vi "EXCOM_25_no_count.vi"(0 "VISA resource name":refnum<visa-resource-name>, 4 "error in":errorcluster) -> (5 "OK Done":bool, 6 "HA":dbl format="%<%H:%M:%S%0u>t", 7 "Q String":string, 8 "RA":dbl format="%<%H:%M:%S%0u>t", 9 "Rotateur":dbl format="%.2f", 10 "DEC":dbl format="%<%H:%M:%S%0u>t", 11 "Dome":dbl format="%.2f", 12 "Epoque":dbl format="%.2f", 13 "Focus":dbl format="%.2f", 14 "VISA resource name dup":refnum<visa-resource-name>, 15 "Masse d'air":dbl format="%.2f", 16 "Temps Sidéral":dbl format="%<%H:%M:%S%0u>t", 17 "Temps Universel":dbl format="%<%H:%M:%S%0u>t", 18 "Année":dbl format="%.2f", 19 "error out":errorcluster)   [LabVIEW 2011]
panel:
  # "3 = COM4"
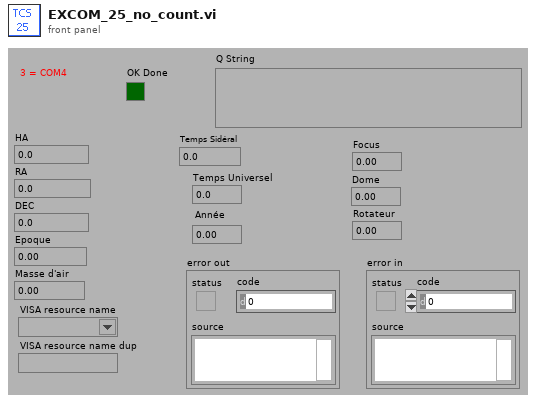
[diagram p1: front panel]
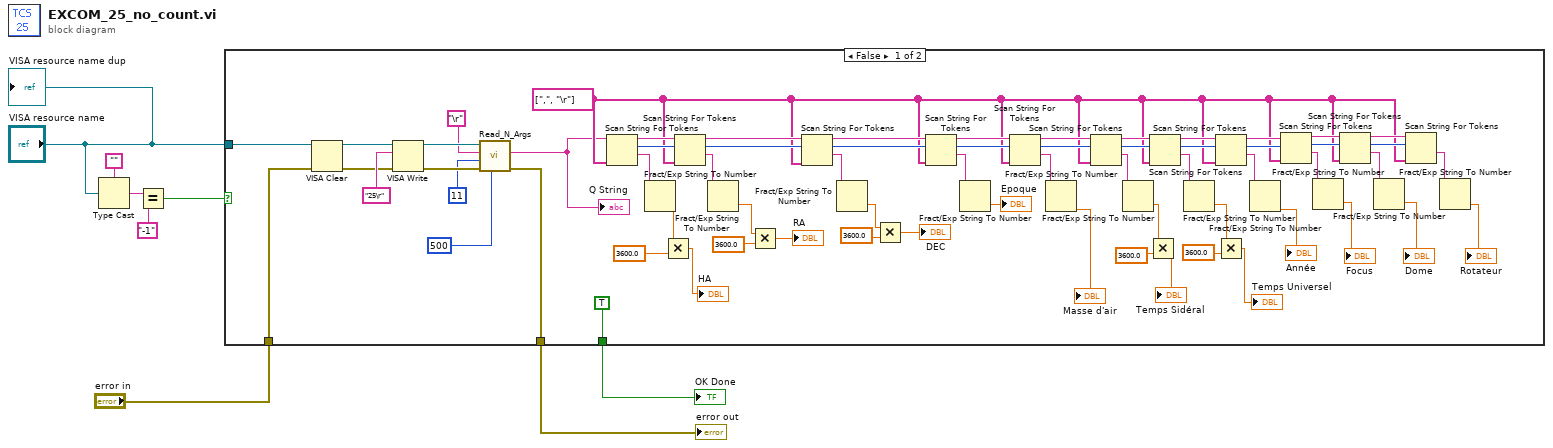
[diagram p0: block diagram]
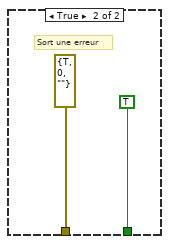
[diagram p2: hidden frame]
diagram:
  n1 = Type Cast(type="", x="VISA resource name") -> (*(type *) &x=w7:string)
  n2 = Equal?(x=w7, y="-1") -> (x = y?=w5:bool)
  n3 = case shown="False" w5 {
    tunnel: "VISA resource name" -> [w12 _]
    tunnel: [TRUE ("OK Done") TRUE ("OK Done")] -> w3
    tunnel: [w19 errorcluster {"status"=TRUE, "code"=0, "source"=""} ("error out")] -> w2
    tunnel: "error in" -> [w10 _]
    frame False {
      w23 = string[] [",", "\r"] ("delimiters (\\s,\\t,\\r,\\n)")
      n4 = VISA Clear(VISA resource name=w12, error in (no error)=w10) -> (VISA resource name out=w11:refnum<visa-resource-name>, error out=w9:errorcluster)
      n5 = VISA Write(VISA resource name=w11, write buffer="25\r" ("String to Send"), error in (no error)=w9) -> (VISA resource name out=w17:refnum<visa-resource-name>, error out=w18:errorcluster)  [unwired: 1 out]
      n6 = call "Read_N_Args.vi"("Delay (ms)"=u32 500, "Error IN"=w18, "Nb_Args"=11, "Arg_Char"="\r", "VRN IN"=w17) -> ("Error OUT"=w19:errorcluster, "Answer"=w20:string)  [unwired: 3 in, 2 out]
      "Q String" <- w20
      n7 = Scan String For Tokens(6:w23, 9:w20) -> (1:w66:string, 2:w67:i32, 3:w68:string)  [unwired: 4 in, 1 out]
      n8 = Fract/Exp String To Number(string=w66) -> (number=w65:dbl)  [unwired: 3 in, 1 out]
      n9 = Multiply(x=w65, y=3600.0) -> (x*y=→"HA":dbl)
      n10 = Scan String For Tokens(6:w23, 8:w67, 9:w68) -> (1:w24:string, 2:w70:i32, 3:w69:string)  [unwired: 3 in, 1 out]
      n11 = Fract/Exp String To Number(string=w24) -> (number=w57:dbl)  [unwired: 3 in, 1 out]
      n12 = Multiply(x=w57, y=3600.0) -> (x*y=→"RA":dbl)
      n13 = Scan String For Tokens(6:w23, 8:w70, 9:w69) -> (1:w60:string, 2:w72:i32, 3:w71:string)  [unwired: 3 in, 1 out]
      n14 = Fract/Exp String To Number(string=w60) -> (number=w55:dbl)  [unwired: 3 in, 1 out]
      n15 = Multiply(x=w55, y=3600.0) -> (x*y=→"DEC":dbl)
      n16 = Scan String For Tokens(6:w23, 8:w72, 9:w71) -> (1:w59:string, 2:w74:i32, 3:w73:string)  [unwired: 3 in, 1 out]
      n17 = Fract/Exp String To Number(string=w59) -> (number=→"Epoque":dbl)  [unwired: 3 in, 1 out]
      n18 = Scan String For Tokens(6:w23, 8:w74, 9:w73) -> (1:w58:string, 2:w26:i32, 3:w45:string)  [unwired: 3 in, 1 out]
      n19 = Fract/Exp String To Number(string=w58) -> (number=→"Masse d'air":dbl)  [unwired: 3 in, 1 out]
      n20 = Scan String For Tokens(6:w23, 8:w26, 9:w45) -> (1:w50:string, 2:w48:i32, 3:w49:string)  [unwired: 3 in, 1 out]
      n21 = Fract/Exp String To Number(string=w50) -> (number=w53:dbl)  [unwired: 3 in, 1 out]
      n22 = Multiply(x=w53, y=3600.0) -> (x*y=→"Temps Sidéral":dbl)
      n23 = Scan String For Tokens(6:w23, 8:w48, 9:w49) -> (1:w51:string, 2:w46:i32, 3:w47:string)  [unwired: 3 in, 1 out]
      n24 = Fract/Exp String To Number(string=w51) -> (number=w54:dbl)  [unwired: 3 in, 1 out]
      n25 = Scan String For Tokens(6:w23, 8:w46, 9:w47) -> (1:w52:string, 2:w25:i32, 3:w35:string)  [unwired: 3 in, 1 out]
      n26 = Multiply(x=w54, y=3600.0) -> (x*y=→"Temps Universel":dbl)
      n27 = Fract/Exp String To Number(string=w52) -> (number=→"Année":dbl)  [unwired: 3 in, 1 out]
      n28 = Scan String For Tokens(6:w23, 8:w25, 9:w35) -> (1:w38:string, 2:w40:i32, 3:w39:string)  [unwired: 3 in, 1 out]
      n29 = Fract/Exp String To Number(string=w38) -> (number=→"Focus":dbl)  [unwired: 3 in, 1 out]
      n30 = Scan String For Tokens(6:w23, 8:w40, 9:w39) -> (1:w37:string, 2:w42:i32, 3:w41:string)  [unwired: 3 in, 1 out]
      n31 = Fract/Exp String To Number(string=w37) -> (number=→"Dome":dbl)  [unwired: 3 in, 1 out]
      n32 = Scan String For Tokens(6:w23, 8:w42, 9:w41) -> (1:w36:string)  [unwired: 3 in, 3 out]
      n33 = Fract/Exp String To Number(string=w36) -> (number=→"Rotateur":dbl)  [unwired: 3 in, 1 out]
    }
    frame True {
      # "Sort une erreur"
    }
  }
  "OK Done" <- w3
  "error out" <- w2
  "VISA resource name dup" <- "VISA resource name"
